vi "svfa_Check Data Valid [FFT subset] (1 Ch).vi"(0 "signal":waveform(dbl), 2 "restart averaging (F)":bool, 7 "window":T3=1 items=["None"=0, "Hanning"=1, "Hamming"=2, "Blackman-Harris"=3, "Exact Blackman"=4, "Blackman"=5, "Flat Top"=6, "4 Term B-Harris "=7, "7 Term B-Harris"=8, "Low Sidelobe"=9, "Force"=64, "Exponential"=65, "Blackman Nuttall"=11, "Triangle"=30, "Bartlett-Hanning"=31, "Bohman"=32, "Parzen"=33, "Welch"=34, "Kaiser"=60, "Dolph-Chebyshev"=61, "Gaussian"=62], 9 "averaging parameters":T2={"averaging mode"=enum."No averaging", "weighting mode"=enum."Linear", "number of averages"=10, "linear mode"=enum."Auto restart"}, 11 "error in (no error)":errorcluster, 12 "frequency range in":T1={"start frequency"=20.0, "stop frequency"=20000.0} {"stop frequency" format="%.2f"; "start frequency" format="%.2f"}) -> (3 "restart averaging":bool, 4 "dup signal":waveform(dbl), 8 "window":u16(ring)=1 items=["None "=0, "Hanning"=1, "Hamming"=2, "Blackman-Harris"=3, "Exact Blackman"=4, "Blackman"=5, "Flat Top"=6, "4 Term B-Harris "=7, "7 Term B-Harris"=8, "Low Sidelobe"=9, "Force - Exponential"=10, "Gaussian"=62], 10 "dup averaging parameters":T2={"averaging mode"=enum."No averaging", "weighting mode"=enum."Linear", "number of averages"=10, "linear mode"=enum."Auto restart"}, 14 "frequency range out":T1={"start frequency"=20.0, "stop frequency"=20000.0} {"stop frequency" format="%.2f"; "start frequency" format="%.2f"}, 15 "error out":errorcluster)   [LabVIEW 2017]
uses:
  <vilib>/addons/_NISVFA/_Shared subVIs/Controls/svc_Window.ctl
  <vilib>/addons/_NISVFA/_Shared subVIs/Common/svc_Check for Waveform Parameter Continuity (no state).vi
  <vilib>/addons/_NISVFA/_Shared subVIs/Common/svc_Get SV Channel Info.vi
  <vilib>/addons/_NISVFA/_Shared subVIs/Common/svc_Engineering Units to Unit Label.vi
  <vilib>/addons/_NISVFA/_Shared subVIs/Common/svc_Unit Label to Engineering Units.vi
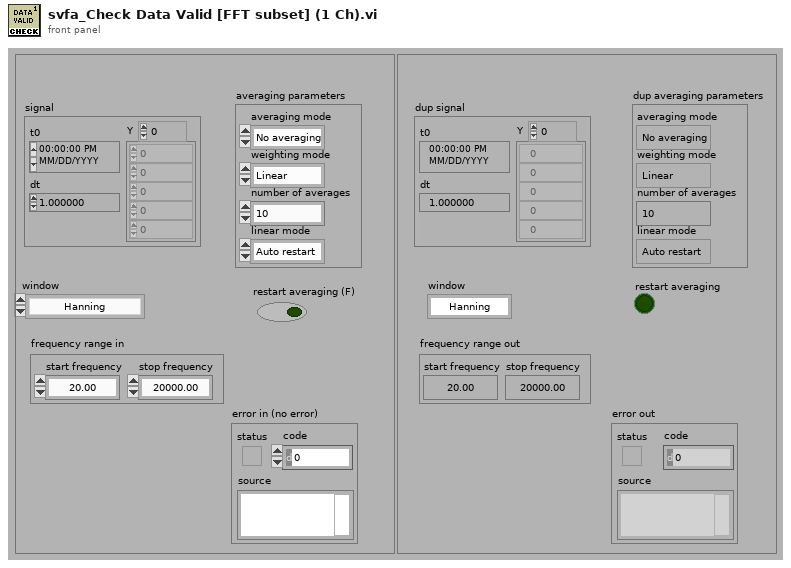
[diagram p1: front panel]
types:
  T1 = cluster{"start frequency":dbl, "stop frequency":dbl}
  T2 = cluster{"averaging mode":enum16{"No averaging", "Vector averaging", "RMS averaging", "Peak hold"}, "weighting mode":enum16{"Linear", "Exponential"}, "number of averages":u32, "linear mode":enum16{"One shot", "Auto restart"}}
  T3 = typedef "svc_Window.ctl" = u32
  T4 = cluster{"dt":bool, "t0 continuity":bool, "array length":bool, "channel info":bool, "name":bool}
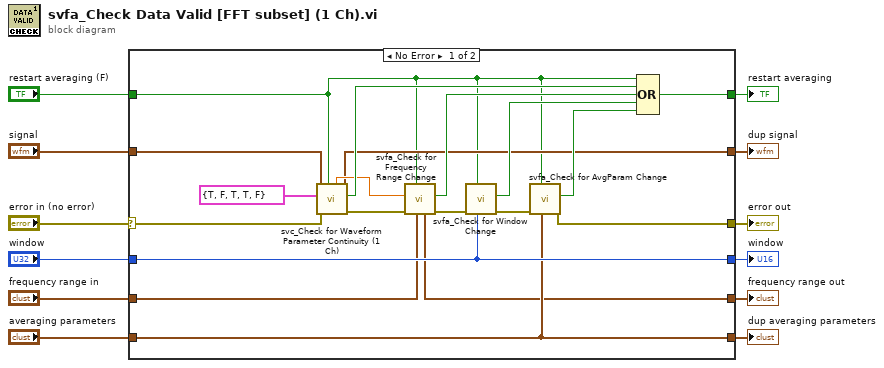
[diagram p0: block diagram]
diagram:
  n1 = case shown="No Error" "error in (no error)" {
    selector: "error in (no error)" -> [w15 w37]
    tunnel: [w13 w37] -> w11
    tunnel: "signal" -> [w19 w35]
    tunnel: "window" -> [w31 w36]
    tunnel: "restart averaging (F)" -> [w14 w32]
    tunnel: [w17 w35] -> w9
    tunnel: [w31 w36] -> w7
    tunnel: "frequency range in" -> [w28 w34]
    tunnel: "averaging parameters" -> [w30 w33]
    tunnel: [w30 w33] -> w4
    tunnel: [w29 w34] -> w3
    tunnel: [w16 w32] -> w1
    frame No Error {
      n2 = call <vilib>:"svc_Check for Waveform Parameter Continuity (1 Ch).vi"("restart averaging (F)"=w14, "error in (no error)"=w15, "checks for channel parameter change"=T4 {"dt"=TRUE, "t0 continuity"=FALSE, "array length"=TRUE, "channel info"=TRUE, "name"=FALSE}, "scaled signal [EU]"=w19) -> ("error out"=w25:errorcluster, "waveform parameter changed"=w20:bool, "dup scaled signal [EU]"=w17:waveform(dbl), "dt"=w18:dbl)  [unwired: 2 in, 2 out]
      n3 = call <vilib>:"svfa_Check for Frequency Range Change.vi"("frequency range in"=w28, "restart averaging (F)"=w14, "error in (no error)"=w25, "dt"=w18) -> ("error out"=w24:errorcluster, "Param_has_changed"=w23:bool, "frequency range out"=w29:T1)  [unwired: 5 in]
      n4 = call <vilib>:"svfa_Check for Window Change.vi"("window"=w31, "restart averaging (F)"=w14, "error in (no error)"=w24) -> ("error out"=w26:errorcluster, "parameter has changed"=w27:bool)  [unwired: 7 in]
      n5 = call <vilib>:"svfa_Check for AvgParam Change.vi"("averaging parameters"=w30, "restart averaging (F)"=w14, "error in (no error)"=w26) -> ("error out"=w13:errorcluster, "parameter has changed"=w22:bool)  [unwired: 7 in]
      n6 = Compound Arithmetic op=OR(w14, w20, w23, w27, w22) -> (w16:bool)
    }
    frame Error {
    }
  }
  "error out" <- w11
  "dup signal" <- w9
  "window" <- w7
  "dup averaging parameters" <- w4
  "frequency range out" <- w3
  "restart averaging" <- w1
